vi "Error Converter (ErrCode or Status).vi"(8 "error in (no error)":errorcluster, 11 "error code":i32) -> (0 "error out":errorcluster)   [LabVIEW 2012, in "KLB.lvlib"]
doc: "wire KLB stack return to error code\n\nswitch (error)\n {\n case 2:\n printf(\"Error during BZIP compression of one of the blocks\");\n break;\n case 5:\n printf(\"Error generating the output file in the specified location\");\n break;\n default:\n printf(\"Error writing the image\");\n}"
uses:
  KLB.lvlib
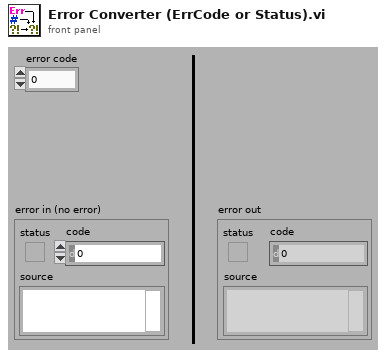
[diagram p1: front panel]
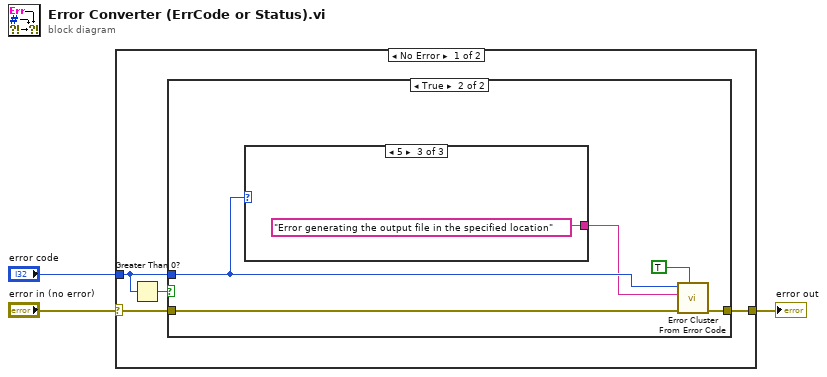
[diagram p0: block diagram]
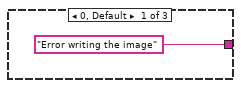
[diagram p3: hidden frame]
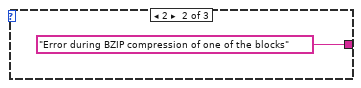
[diagram p4: hidden frame]
diagram:
  n1 = case shown="No Error" "error in (no error)" {
    selector: "error in (no error)" -> [w6 w17]
    tunnel: [w4 w17] -> w2
    tunnel: "error code" -> [w5 _]
    frame No Error {
      n2 = Greater Than 0?(x=w5) -> (x > 0?=w7:bool)
      n3 = case shown="True" w7 {
        tunnel: w6 -> [w8 w13]
        tunnel: w5 -> [_ w10]
        tunnel: [w8 w12] -> w4
        frame False {
        }
        frame True {
          n4 = case shown="5" w10 {
            tunnel: ["Error writing the image" "Error during BZIP compression of one of the blocks" "Error generating the output file in the specified location"] -> w9
            frame 0, Default {
            }
            frame 2 {
            }
            frame 5 {
            }
          }
          n5 = call <vilib>:"Error Cluster From Error Code.vi"("show call chain? (False)"=TRUE, "error in (no error)"=w13, "error message (\"\")"=w9, "error code (0)"=w10) -> ("error out"=w12:errorcluster)  [unwired: 5 in]
        }
      }
    }
    frame Error {
    }
  }
  "error out" <- w2
